vi "Convert Pixels To Picture.vi"(11 "Pixel Data in":u32[][](array[numeric])) -> (2 "Present Time [s]":dbl format="%.1p", 3 "2D Picture":picture)   [LabVIEW 2022 SP3, in "Utility.lvlib"]
uses:
  d601d993-a776-4dc8-89c7-357d8398c88c.vi
  7816d0d6-8e4d-41a2-85ac-ed82f1435763.vi
  <vilib>/Utility/High Resolution Relative Seconds.vi
  <vilib>/picture/picture.llb/Draw True-Color Pixmap.vi
  Utility.lvlib
panel:
  # "(0,0)"
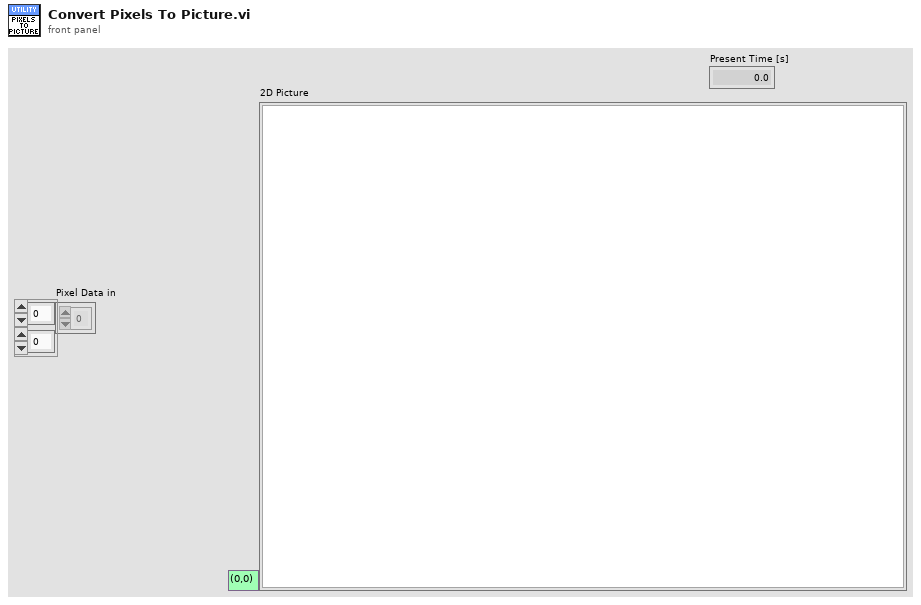
[diagram p1: front panel]
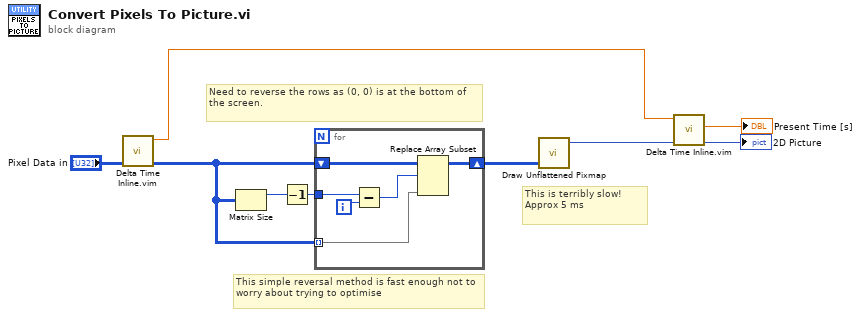
[diagram p0: block diagram]
diagram:
  # "Need to reverse the rows as (0, 0) is at the bottom of the screen."
  # "This simple reversal method is fast enough not to worry about trying to optimise"
  # "This is terribly slow!\nApprox 5 ms"
  n1 = call "Delta Time Inline.vim"("value in"="Pixel Data in") -> ("value out"=w7:u32[][], "Relative Seconds out [s]"=w5:dbl)  [unwired: 8 in, 1 out]
  n2 = Matrix Size(0:w7) -> (1:w2:i32)  [unwired: 1 out]
  n3 = Decrement(x=w2) -> (x-1=w1:i32)
  n4 = for {
    tunnel: w7 -> [w11] mode=indexing
    shift-right: [w10] -> w9
    shift-left: w7 -> [w15]
    tunnel: w1 -> [w14]
    i -> [w13]
    n5 = Subtract(x=w14, y=w13) -> (x-y=w12:i32)
    n6 = Replace Array Subset(array=w15, new element=w11, index (row)=w12) -> (w10:u32[][])  [unwired: 1 in]
  }
  n7 = call-poly <vilib>:"Draw Unflattened Pixmap.vi"("data (RGB format)"=w9) -> ("new picture"=w3:picture)  [unwired: 8 in]
  n8 = call "Delta Time Inline.vim"("value in"=w3, "Relative Seconds in [s]"=w5) -> ("value out"=→"2D Picture":picture, "Delta Time [s]"=→"Present Time [s]":dbl)  [unwired: 7 in, 1 out]
